vi "LEP_RV_LaunchStartInit.vi"(8 "error in (no error)":errorcluster, 11 "buildSpec ID":string) -> (0 "error out":errorcluster)   [LabVIEW 2011]
doc: "Download and execute built VxWorks downloadable module and attach the LabVIEW Embedded debuger."
panel:
  out "output cluster":T1
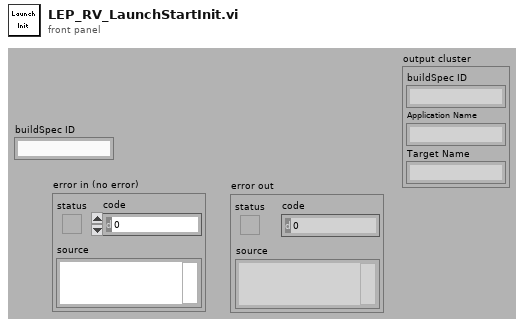
[diagram p1: front panel]
types:
  T1 = cluster{"buildSpec ID":string, "Application Name":string, "Target Name":string}
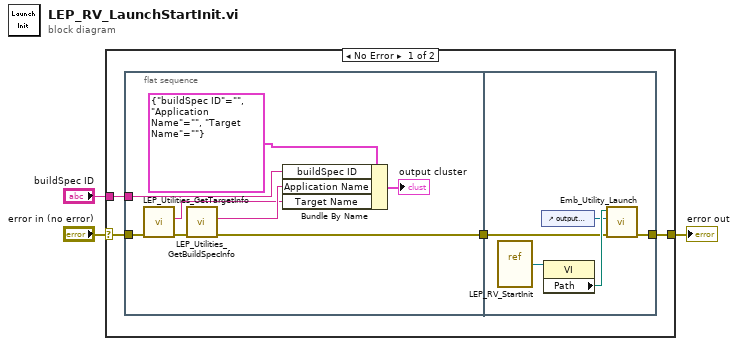
[diagram p0: block diagram]
diagram:
  n1 = case shown="No Error" "error in (no error)" {
    selector: "error in (no error)" -> [w7 w21]
    tunnel: [w5 w21] -> w3
    tunnel: "buildSpec ID" -> [w4 _]
    frame No Error {
      n2 = flat-sequence {
        tunnel: w7 -> [w15]
        tunnel: [w13] -> w6
        tunnel: w4 -> [w11]
        tunnel: w6 -> [w17]
        tunnel: [w16] -> w5
        frame #0 {
          n3 = call <vilib>:"LEP_Utilities_GetTargetInfo.vi"("error in"=w15) -> ("error out"=w14:errorcluster, "display name"=w8:string)  [unwired: 9 out]
          n4 = call <vilib>:"LEP_Utilities_GetBuildSpecInfo.vi"("error in"=w14) -> ("error out"=w13:errorcluster, "display name"=w9:string)  [unwired: 9 out]
          n5 = Bundle By Name(cluster=T1 {"buildSpec ID"="", "Application Name"="", "Target Name"=""}, "buildSpec ID"=w11, "Application Name"=w9, "Target Name"=w8) -> (→"output cluster":T1)
        }
        frame #1 {
          n6 = vi-ref "LEP_RV_StartInit.vi"() -> (w20:refnum<vi>)
          n7 = control-ref of="output cluster"() -> (w18:refnum<vi>)
          n8 = property class="VI"(reference=w20) -> ("Path"=w19:path)  [unwired: 1 in, 2 out]
          n9 = call <vilib>:"Emb_Utility_Launch.vi"("error in"=w17, "parameter cluster"=w18, "vi path"=w19) -> ("error out"=w16:errorcluster)  [unwired: 6 out]
        }
      }
    }
    frame Error {
    }
  }
  "error out" <- w3
